vi "LS330_Read_TEMPS.vi"(6 "error in (no error)":errorcluster, 9 "VISA Refnum in":refnum<visa-resource-name>) -> (0 "error out":errorcluster, 1 "Temp B (K)":dbl, 2 "Temp A (K)":dbl, 3 "VISA Refnum out":refnum<visa-resource-name>)   [LabVIEW 2021]
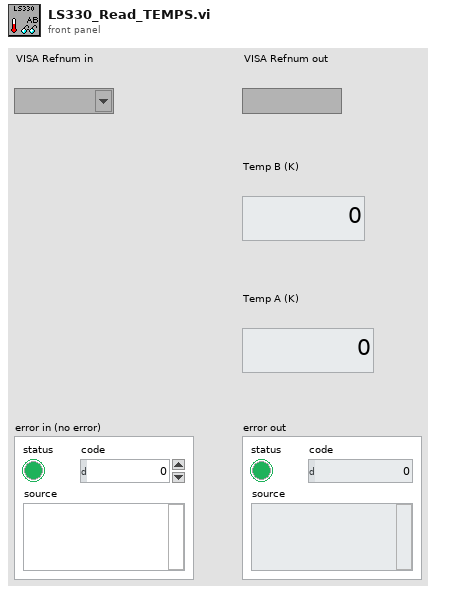
[diagram p1: front panel]
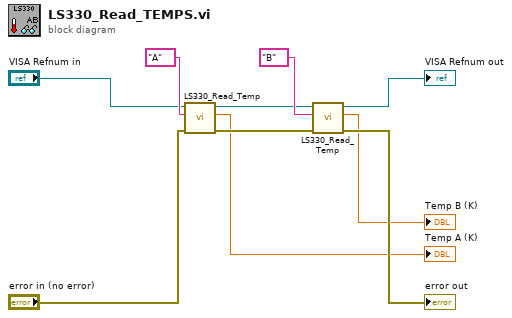
[diagram p0: block diagram]
diagram:
  n1 = call "LS330_Read_Temp.vi"("error in"="error in (no error)", "Channel"="A", "VISA resource name"="VISA Refnum in") -> ("error out"=w6:errorcluster, "Temp (K)"=→"Temp A (K)":dbl, "VISA resource name out"=w4:refnum<visa-resource-name>)  [unwired: 6 in]
  n2 = call "LS330_Read_Temp.vi"("error in"=w6, "Channel"="B", "VISA resource name"=w4) -> ("error out"=→"error out":errorcluster, "Temp (K)"=→"Temp B (K)":dbl, "VISA resource name out"=→"VISA Refnum out":refnum<visa-resource-name>)  [unwired: 6 in]
